vi "Data_base_client.vi"(4 "Average Sampling freq":sgl=100.0 format="%.1f", 5 "Channels from Client":string[][](array[string])=[["Data Base:Measurement:Type", "LDA & Cw"], ["Data Base:Position:No of Inst", "2"], ["Data Base:Position:X1", "-60"], ["Data Base:Position:X2", ""], ["Data Base:Position:Y1", "2"], ["Data Base:Position:Y2", "0.00"], ["Data Base:Position:Z1", "0.00"], ["Data Base:Position:Z2", "2.00"]], 6 "Average Meas Time (min)":dbl=100.0 format="%.1f", 7 "End time":dbl, 8 "Start time":dbl, 9 "Results File Pathname":path, 10 "Raw Data Pathname":path) -> (1 "spreadsheet string":string, 2 "Channel values":string[](array[string]), 3 "Channel names":string[](array[string]))   [LabVIEW 2020]
doc: "This is an example of using features of the VI Server as a client. It shows how you might browse from one or more applications that may be exporting data from one or more data stations. \n\nThe example shows how to query a server for its list of exported VIs, how to get references to the VIs, and how call them with the Call By Reference function."
uses:
  Anemometry/Anemometry Sub Vis/Globals/Preference_global.vi
panel:
  out "Iterations":i32
  in  "Data Base server type":refnum<vi>
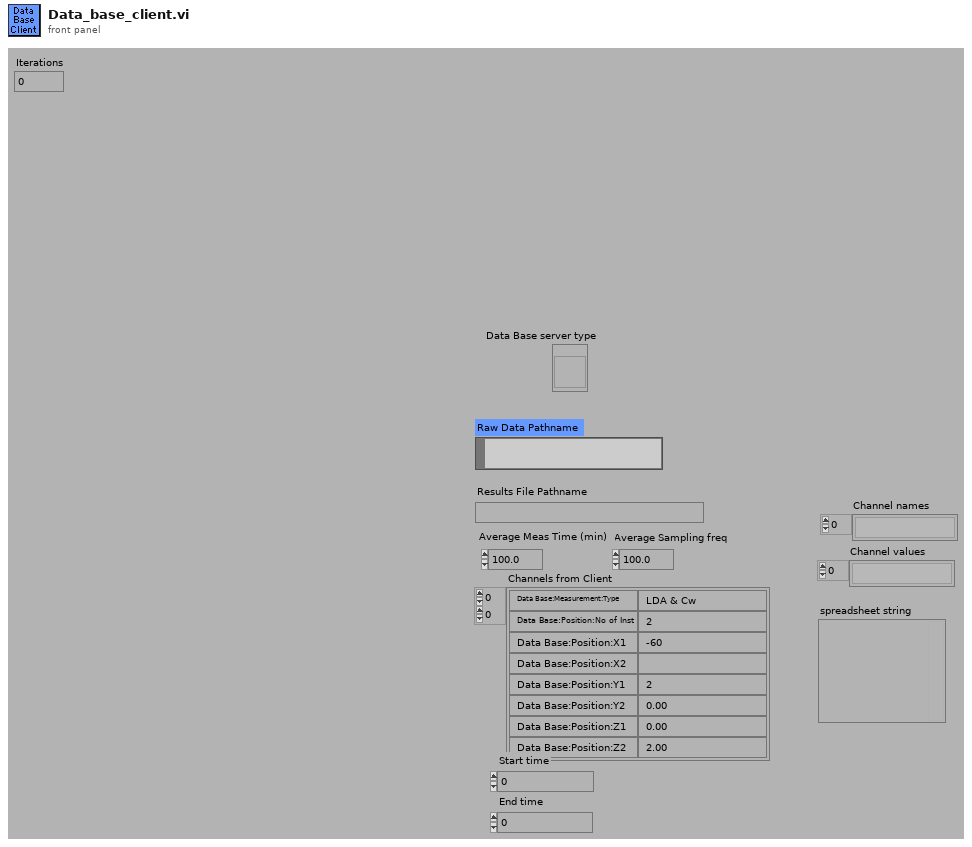
[diagram p1: front panel]
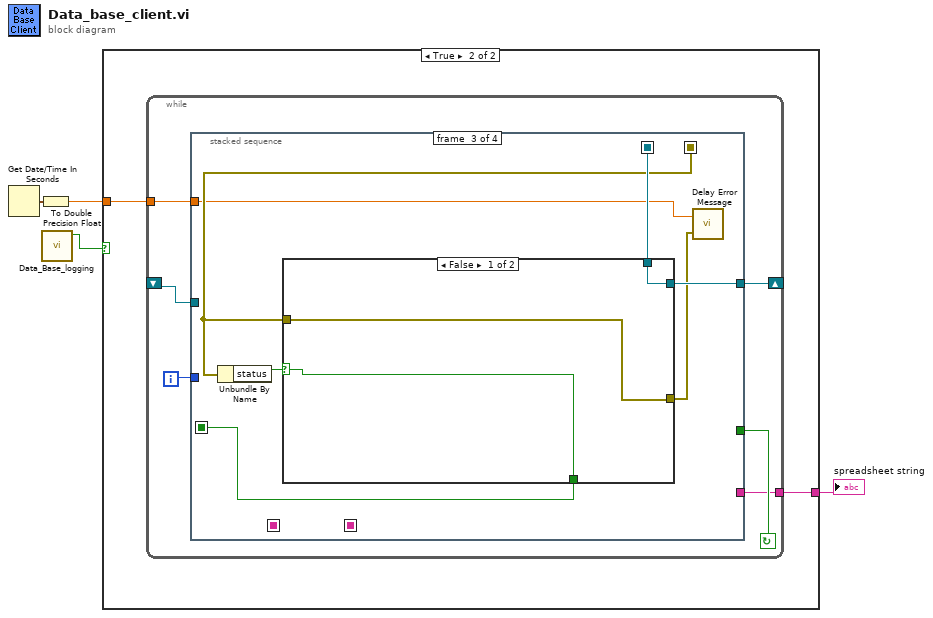
[diagram p0: block diagram]
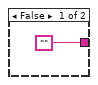
[diagram p2: hidden frame]
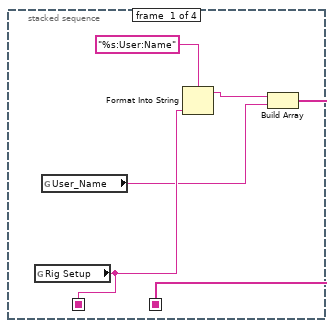
[diagram p3: hidden frame]
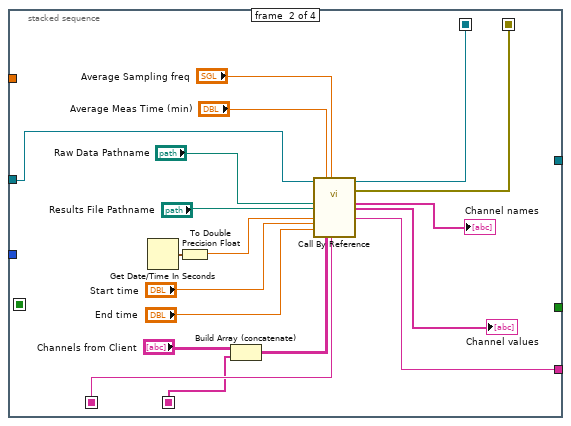
[diagram p4: hidden frame]
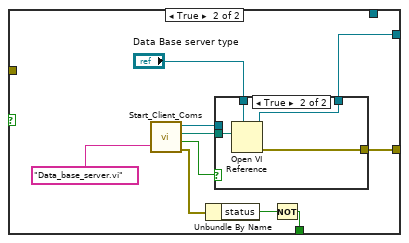
[diagram p5: hidden frame]
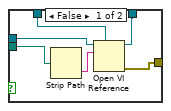
[diagram p6: hidden frame]
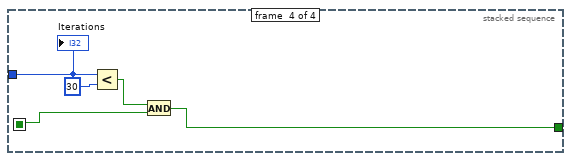
[diagram p7: hidden frame]
diagram:
  n1 = Get Date/Time In Seconds() -> (seconds since 1Jan1904=w2:timestamp)
  n2 = To Double Precision Float(number=w2) -> (double precision float=w1:dbl)
  n3 = call "Data_Base_logging.vi"() -> ("Logging On?"=w3:bool)  [unwired: 4 out]
  n4 = case shown="True" w3 {
    tunnel: ["" w7] -> w4
    tunnel: w1 -> [_ w6]
    frame False {
    }
    frame True {
      n5 = while {
        tunnel: [w9] -> w7
        shift-left: _ -> [w13]
        shift-right: [w12] -> _
        tunnel: w6 -> [w8]
        i -> [w11]
        stop <- w10 continue-if-true
        n6 = stacked-sequence {
          seq-local: [_ w29 _ _] -> [_ _ w42 _]
          seq-local: [_ w28 _ _] -> [_ _ w40 _]
          seq-local: [_ _ w37 _] -> [_ _ _ w68]
          seq-local: [w18 _ _ _] -> [_ w22 _ _]
          seq-local: [w14 _ _ _] -> [_ w19 _ _]
          tunnel: w13 -> [_ w30 _ _]
          tunnel: [_ _ w43 _] -> w12
          tunnel: w11 -> [_ _ _ w69]
          tunnel: [_ _ _ w67] -> w10
          tunnel: [_ w25 _ _] -> w9
          tunnel: w8 -> [_ _ w39 _]
          frame #0 {
            n7 = global read "Preference_global.vi" "Rig Setup"() -> (w18:string)
            n8 = global read "Preference_global.vi" "User_Name"() -> (w15:string)
            n9 = Format Into String(format string="%s:User:Name", w18) -> (resulting string=w16:string)  [unwired: 2 in, 1 out]
            n10 = Build Array(w16, w15) -> (w14:string[])
          }
          frame #1 {
            n11 = Get Date/Time In Seconds() -> (seconds since 1Jan1904=w23:timestamp)
            n12 = To Double Precision Float(number=w23) -> (double precision float=w32:dbl)
            n13 = Build Array (concatenate)("Channels from Client", w19) -> (w20:string[][])
            n14 = call-by-ref "?"(reference=w30, "Raw Data Pathname"="Raw Data Pathname", "Results File Pathname"="Results File Pathname", "Clients time"=w32, "Start time"="Start time", "End time"="End time", "Average Meas Time (min)"="Average Meas Time (min)", "Channels from Client"=w20, "Average Sampling freq"="Average Sampling freq", "Rig Name"=w22) -> (reference out=w29:refnum<vi>, error out=w28:errorcluster, "Channel names"=→"Channel names":string[], "Channel values"=→"Channel values":string[], "spreadsheet string"=w25:string)  [unwired: 9 in]
          }
          frame #2 {
            n15 = Unbundle By Name(w40) -> ("status"=w41:bool)
            n16 = case shown="False" w41 {
              selector: w41 -> [w44 _]
              tunnel: [w46 w52] -> w43
              tunnel: w42 -> [w46 _]
              tunnel: [w45 w50] -> w38
              tunnel: w40 -> [w45 _]
              tunnel: [w44 w47] -> w37
              frame False {
              }
              frame True {
                n17 = call "Start_Client_Coms.vi"("VI name to run on server"="Data_base_server.vi") -> ("LabVIEW application reference"=w54:refnum<vi>, "Checked VI name"=w55:path, "Local Call"=w53:bool, "Error cluster"=w48:errorcluster)  [unwired: 1 in]
                n18 = Unbundle By Name(w48) -> ("status"=w49:bool)
                n19 = case shown="True" w53 {
                  tunnel: [w58 w66] -> w52
                  tunnel: "Data Base server type" -> [w59 w65]
                  tunnel: w55 -> [w61 w64]
                  tunnel: w54 -> [w60 _]
                  tunnel: [w57 w63] -> w50
                  frame False {
                    n20 = Strip Path(path=w61) -> (name=w62:string)  [unwired: 1 out]
                    n21 = Open VI Reference(type specifier VI Refnum (for type only)=w59, application reference (local)=w60, vi path=w62) -> (vi reference=w58:refnum<vi>, error out=w57:errorcluster)  [unwired: 1 in, 2 out]
                  }
                  frame True {
                    n22 = Open VI Reference(type specifier VI Refnum (for type only)=w65, vi path=w64) -> (vi reference=w66:refnum<vi>, error out=w63:errorcluster)  [unwired: 1 in, 3 out]
                  }
                }
                n23 = Not(x=w49) -> (.not. x?=w47:bool)
              }
            }
            n24 = call "Delay Error Message.vi"("error in (no error)"=w38, "Seconds since 1904"=w39) -> ()  [unwired: 2 in]
          }
          frame #3 {
            n25 = Less?(x=w69, y=30) -> (x < y?=w71:bool)
            n26 = And(x=w71, y=w68) -> (x .and. y?=w67:bool)
            "Iterations" <- w69
          }
        }
      }
    }
  }
  "spreadsheet string" <- w4
